vi "set_item.vi"(6 "close_item? (true)":bool=TRUE, 8 "error in (no error)":errorcluster, 9 "Item":refnum<class "Item.lvclass">, 10 "item_name":string, 11 "Doc in":refnum<class "Doc.lvclass">) -> (0 "error out":errorcluster, 3 "Doc out":refnum<class "Doc.lvclass">)   [LabVIEW 2020, in "toml_edit.lvlib" / "Doc.lvclass"]
uses:
  Doc.lvclass
  Item/Item.lvclass
  Doc.lvclass/Doc.ctl
  Item/Item.lvclass/Item.ctl
  dragon_toml_64.dll
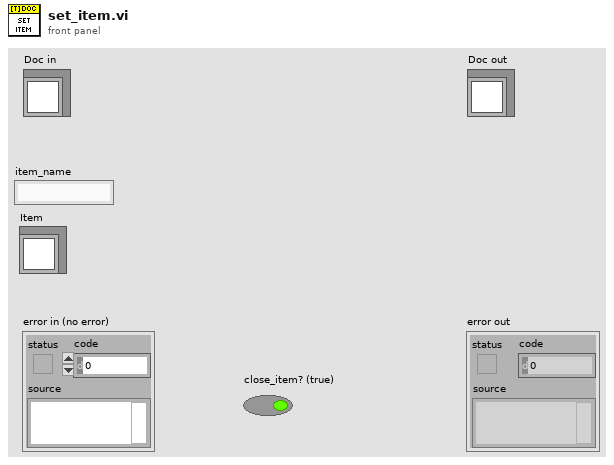
[diagram p1: front panel]
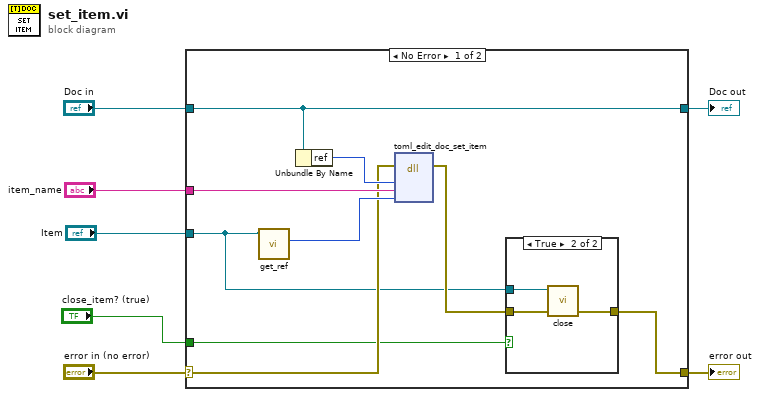
[diagram p0: block diagram]
diagram:
  n1 = case shown="No Error" "error in (no error)" {
    selector: "error in (no error)" -> [w12 w22]
    tunnel: [w11 w22] -> w6
    tunnel: [w16 w21] -> w4
    tunnel: "Doc in" -> [w16 w21]
    tunnel: "Item" -> [w9 _]
    tunnel: "item_name" -> [w13 _]
    tunnel: "close_item? (true)" -> [w8 _]
    frame No Error {
      n2 = call "get_ref.vi"("Item in"=w9) -> ("ref"=w15:u64)  [unwired: 10 in]
      n3 = Unbundle By Name(w16) -> ("ref"=w14:u64)
      n4 = dll-call lib="C:/Users/JamesMcNally/Documents/toml-edit-labview/lv_src/dragon_toml_*.*" fn="toml_edit_doc_set_item"(error in=w12, "table_ref"=w14, "item_name"=w13, "item_ref"=w15) -> (error out=w10:errorcluster)  [unwired: 6 in, 1 out]
      n5 = case shown="True" w8 {
        tunnel: w10 -> [w17 w20]
        tunnel: [w17 w19] -> w11
        tunnel: w9 -> [_ w18]
        frame False {
        }
        frame True {
          n6 = call "close.vi"("error in (no error)"=w20, "Item in"=w18) -> ("error out"=w19:errorcluster)  [unwired: 9 in]
        }
      }
    }
    frame Error {
    }
  }
  "error out" <- w6
  "Doc out" <- w4
